vi "Combined_file_Panel.vi"(7 "Show panel ?":bool, 10 "Output filename":path=path "/G3_3 HD/Users/Paul/New Disp DB file") -> (0 "Only Plotted data?":bool, 1 "Include Empty Rows? Out":bool, 2 "Give Audit Channels Out":bool, 3 "Output filename Out":path=path "/G3_3 HD/Users/Paul/New Disp DB file")   [LabVIEW 2014]
panel:
  in  "Include Empty Rows?":bool
  in  "Give Audit Channels":bool
  in  "OK Button":bool
  in  "Row Selector":i32(listbox)
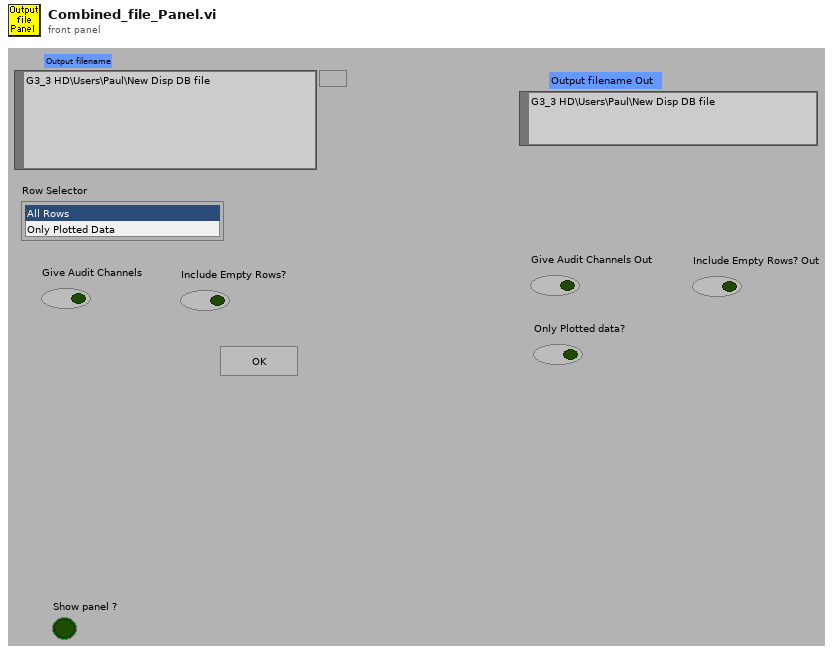
[diagram p1: front panel]
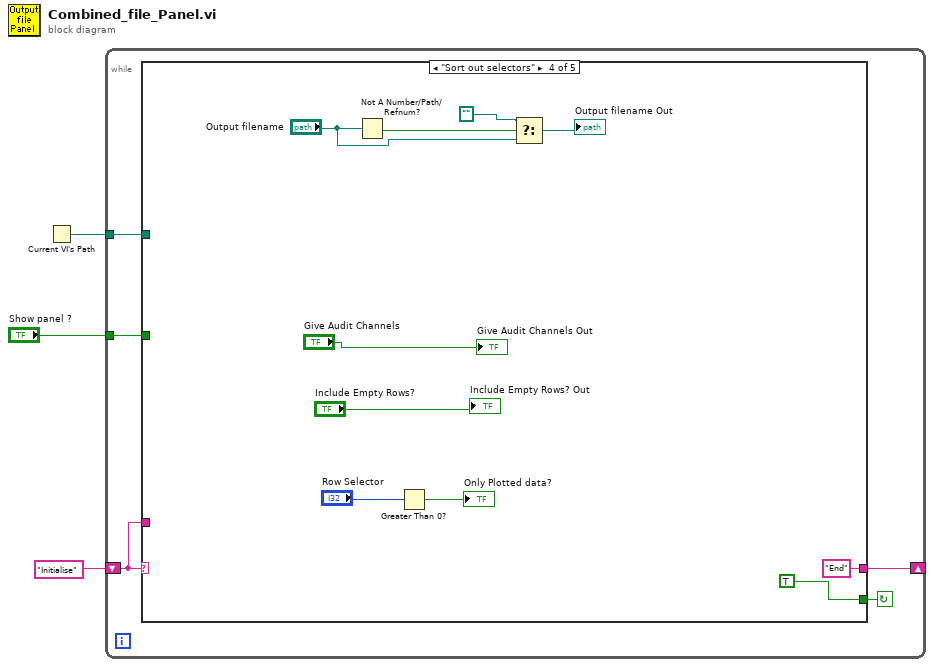
[diagram p0: block diagram]
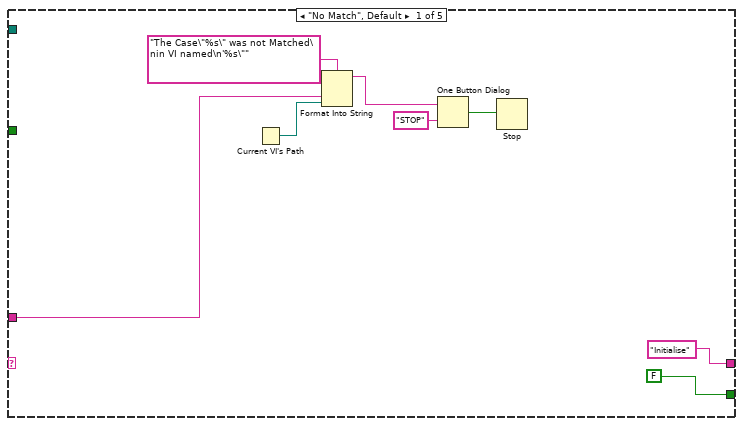
[diagram p2: hidden frame]
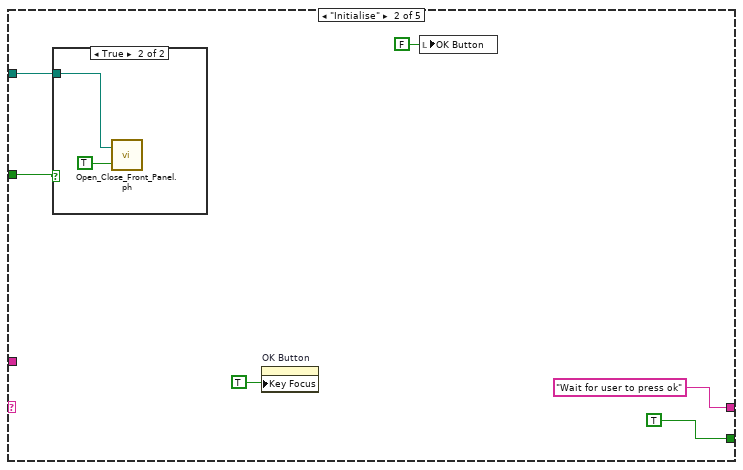
[diagram p3: hidden frame]
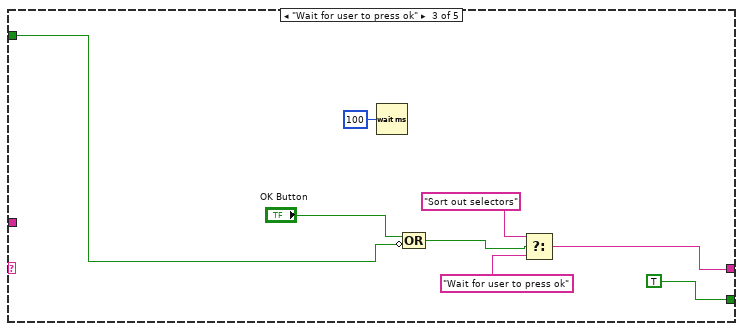
[diagram p5: hidden frame]
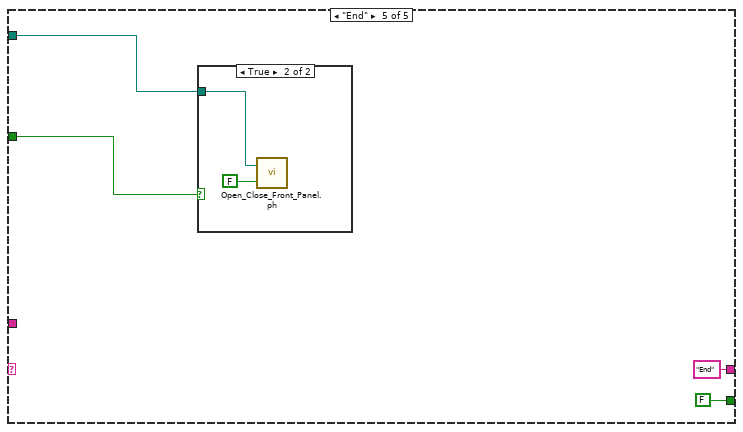
[diagram p6: hidden frame]
diagram:
  n1 = Current VI's Path() -> (path=w1:path)
  n2 = while {
    shift-left: "Initialise" -> [w6]
    shift-right: [w7] -> _
    tunnel: "Show panel ?" -> [w5]
    tunnel: w1 -> [w4]
    stop <- w8 continue-if-true
    n3 = case shown="\"Sort out selectors\"" w6 {
      tunnel: [FALSE TRUE TRUE TRUE FALSE] -> w8
      tunnel: ["Initialise" "Wait for user to press ok" w31 "End" ("t") "End"] -> w7
      tunnel: w6 -> [w11 _ _ _ _]
      tunnel: w5 -> [_ w19 w25 _ w44]
      tunnel: w4 -> [_ w18 _ _ w43]
      frame "No Match", Default {
        n4 = Current VI's Path() -> (path=w10:path)
        n5 = Format Into String(format string="The Case\"%s\" was not Matched\nin VI named\n'%s\"" ("Format String"), w11, w10) -> (resulting string=w14:string)  [unwired: 2 in, 1 out]
        n6 = One Button Dialog(message=w14, button name ("OK")="STOP") -> (true=w12:bool)
        n7 = Stop(stop? (T)=w12) -> ()
      }
      frame "Initialise" {
        n8 = case shown="True" w19 {
          tunnel: w18 -> [_ w24]
          frame False {
          }
          frame True {
            n9 = call "Open_Close_Front_Panel.ph.vi"("Front Panel Window:Open"=TRUE, "VI path"=w24) -> ()  [unwired: 2 out]
          }
        }
        n10 = property on="OK Button" class="Bool (strict)"("Key Focus"=TRUE) -> ()  [unwired: 2 in, 2 out]
        n11 = local write "OK Button"(FALSE ("OK Button")) -> ()
      }
      frame "Wait for user to press ok" {
        n12 = Wait (ms)(milliseconds to wait=u32 100) -> ()  [unwired: 1 out]
        n13 = Compound Arithmetic op=OR("OK Button", invert w25) -> (w26:bool)
        n14 = Select(t="Sort out selectors", s=w26, f="Wait for user to press ok") -> (s? t:f=w31:string)
      }
      frame "Sort out selectors" {
        n15 = Not A Number/Path/Refnum?(number/path/refnum="Output filename") -> (NaN/Path/Refnum?=w39:bool)
        n16 = Greater Than 0?(x="Row Selector") -> (x > 0?=→"Only Plotted data?":bool)
        n17 = Select(t=path "", s=w39, f="Output filename") -> (s? t:f=→"Output filename Out":path)
        "Include Empty Rows? Out" <- "Include Empty Rows?"
        "Give Audit Channels Out" <- "Give Audit Channels"
      }
      frame "End" {
        n18 = case shown="True" w44 {
          tunnel: w43 -> [_ w48]
          frame False {
          }
          frame True {
            n19 = call "Open_Close_Front_Panel.ph.vi"("Front Panel Window:Open"=FALSE, "VI path"=w48) -> ()  [unwired: 2 out]
          }
        }
      }
    }
  }
